vi "MU Calibration Nonius Phase Margin.vi"(8 "error in (no error)":errorcluster, 11 "analyzeResult":T1) -> (0 "error out":errorcluster, 2 "PhaseMargin":i32[](array[numeric]), 3 "Return Value":u64)   [LabVIEW 2017, in "MU_3SL_interface.lvlib"]
uses:
  MU_3SL_interface.lvlib
  handles/CalibrationAnalyzeResultHandle.ctl
  lib/MU_3SL_interface.dll
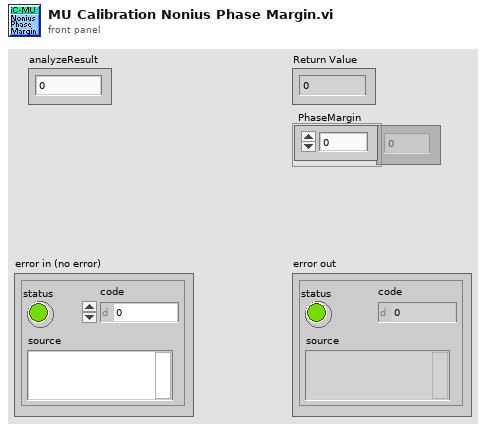
[diagram p1: front panel]
types:
  T1 = typedef "MU_3SL_interface.lvlib/CalibrationAnalyzeResultHandle.ctl" = u64
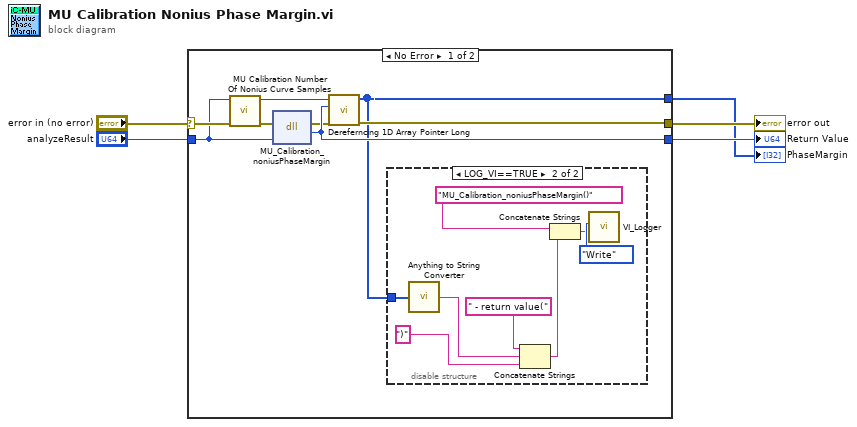
[diagram p0: block diagram]
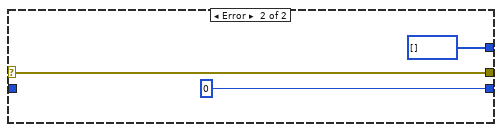
[diagram p3: hidden frame]
diagram:
  n1 = case shown="No Error" "error in (no error)" {
    selector: "error in (no error)" -> [w13 w24]
    tunnel: "analyzeResult" -> [w12 _]
    tunnel: [w7 w24] -> w4
    tunnel: [w10 u64 0 ("return type")] -> w3
    tunnel: [w6 i32[] [] ("Array Data")] -> w1
    frame No Error {
      n2 = call "MU Calibration Number Of Nonius Curve Samples.vi"("error in (no error)"=w13, "CalibrationAnalyzeResult"=w12) -> ("error out"=w11:errorcluster, "NumberOfNoniusCurveSamples"=w8:u64)  [unwired: 8 in]
      n3 = dll-call lib="C:/Users/bes/AppData/Roaming/work/mu_9so/icsubmodules/soft_mu_3sl_master/lv_interface/lib/MU_3SL_interface**.*" fn="MU_Calibration_noniusPhaseMargin"(error in=w11, "analyzeResult"=w12) -> (error out=w9:errorcluster, "PhaseErrorHandle"=w10:u64)  [unwired: 3 in, 1 out]
      n4 = call "Dereferncing 1D Array Pointer Long.vi"("error in (no error)"=w9, "1D Double Array Pointer"=w10, "numberOfSamples"=w8) -> ("error out"=w7:errorcluster, "Array Data"=w6:i32[])  [unwired: 7 in]
      n5 = disable-structure shown="LOG_VI==TRUE" {
        disable-tunnel: w6 -> [_ w15]
        frame condition #0 {
        }
        frame condition #1 (active) {
          n6 = call "Anything to String Converter.vi"("anything"=w15) -> ("String"=w14:string)
          n7 = Concatenate Strings(" - return value(" ("string"), w14, ")" ("string")) -> (w19:string)
          n8 = Concatenate Strings("MU_Calibration_noniusPhaseMargin()" ("Info in"), w19) -> (w18:string)
          n9 = call "VI_Logger.vi"("Action (Read)"=enum16{"Write", "Read"}."Write", "Info in"=w18) -> ()  [unwired: 8 in, 2 out]
        }
      }
    }
    frame Error {
    }
  }
  "error out" <- w4
  "Return Value" <- w3
  "PhaseMargin" <- w1
